vi "Create for Application.vi"(8 "error in (no error)":errorcluster, 11 "Application":refnum<vi>) -> (0 "error out":errorcluster, 3 "CodeCoverage out":refnum<class "Code Coverage.lvclass">)   [LabVIEW 2017, in "Code Coverage.lvclass"]
uses:
  Code Coverage.lvclass
  Code Coverage.lvclass/Code Coverage.ctl
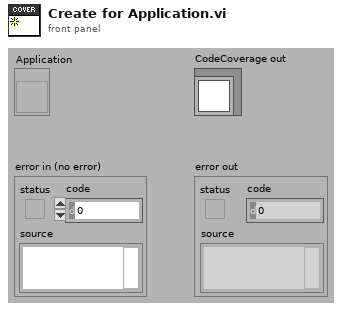
[diagram p1: front panel]
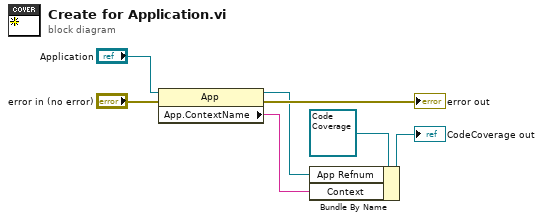
[diagram p0: block diagram]
diagram:
  n1 = property class="App"(reference="Application", error in="error in (no error)") -> (reference out=w2:refnum<vi>, error out=→"error out":errorcluster, "App.ContextName"=w5:string)
  n2 = Bundle By Name(cluster=refnum<class "Code Coverage.lvclass"> refnum ("CodeCoverage in"), "App Refnum"=w2, "Context"=w5) -> (→"CodeCoverage out":refnum<class "Code Coverage.lvclass">)
